vi "PXI Compute Skip Samples.vi"(0 "AO Tasks":T1[](array[typedef]), 7 "AI Tasks":T1[](array[typedef]), 11 "error in (no error)":errorcluster) -> (4 "Skip Samples":i32, 15 "error out":errorcluster)   [LabVIEW 2020]
doc: "Determines the number of AI samples to skip in order to register AO and AI (accounting for the latencies of the 24-bit boards)."
uses:
  Type Defs/Task Struct.ctl
  PXI Globals.vi
panel:
  out "Any 16-bit AI?":bool
  out "Any 16-bit AO?":bool
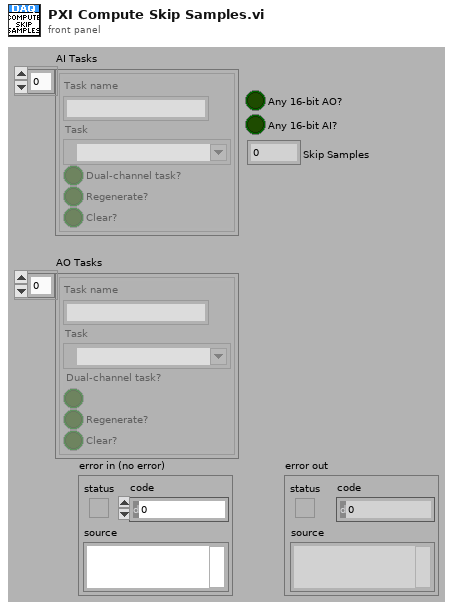
[diagram p1: front panel]
types:
  T1 = typedef "Task Struct.ctl" = cluster{"Task name":string, "Task":refnum<k21>, "Dual-channel task?":bool, "Regenerate?":bool, "Clear?":bool}
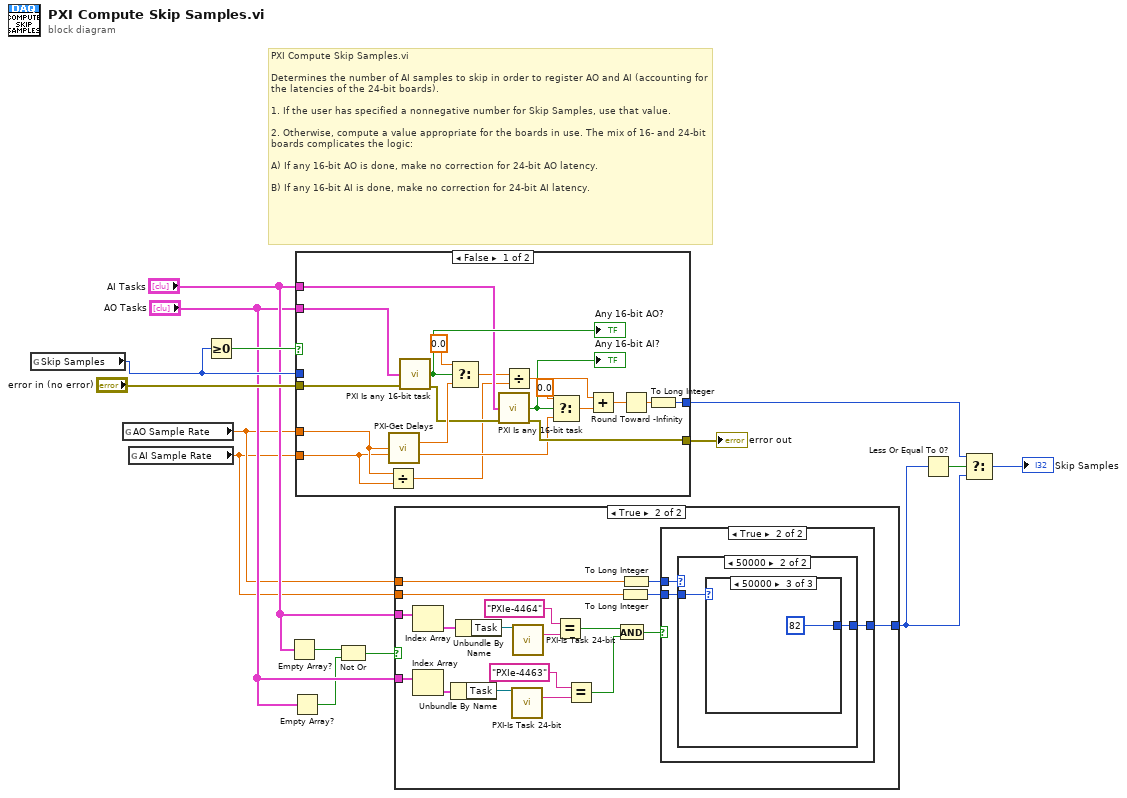
[diagram p0: block diagram]
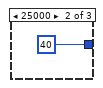
[diagram p6: hidden frame]
diagram:
  # "PXI Compute Skip Samples.vi\n\nDetermines the number of AI samples to skip in order to register AO and AI (accounting for the latencies of the 24-bit boards). \n\n1. If the user has specified a nonnegative number for Skip Samples, use that value. \n\n2. Otherwise, compute a value appropriate for the boards in use. The mix of 16- and 24-bit boards complicates the logic:\n\nA) If any 16-bit AO is done, make no correction for 24-bit AO latency.\n\nB) If any 16-bit AI is done, make no correction for 24-bit AI latency."
  n1 = global read "PXI Globals.vi" "Skip Samples"() -> (w12:i32)
  n2 = global read "PXI Globals.vi" "AO Sample Rate"() -> (w6:dbl)
  n3 = global read "PXI Globals.vi" "AI Sample Rate"() -> (w5:dbl)
  n4 = Greater Or Equal To 0?(x=w12) -> (x >= 0?=w15:bool)
  n5 = Empty Array?(array="AI Tasks") -> (empty?=w9:bool)
  n6 = Empty Array?(array="AO Tasks") -> (empty?=w8:bool)
  n7 = case shown="False" w15 {
    tunnel: "error in (no error)" -> [w16 w37]
    tunnel: [w33 w36] -> w4
    tunnel: [w26 w37] -> w14
    tunnel: w12 -> [_ w36]
    tunnel: "AO Tasks" -> [w32 _]
    tunnel: "AI Tasks" -> [w27 _]
    tunnel: w6 -> [w18 _]
    tunnel: w5 -> [w17 _]
    frame False {
      n8 = Divide(x=w18, y=w17) -> (x/y=w19:dbl)
      n9 = call "PXI-Get Delays.vi"("AO Rate (Samples/s)"=w18, "AI Rate (Samples/s)"=w17) -> ("AO delay (samples)"=w29:dbl, "AI delay (samples)"=w24:dbl)  [unwired: 12 in]
      n10 = call "PXI Is any 16-bit task.vi"("Task Array"=w32, "error in (no error)"=w16) -> ("Any 16-bit task?"=w31:bool, "error out"=w28:errorcluster)  [unwired: 12 in]
      "Any 16-bit AO?" <- w31
      n11 = Select(t=0.0 ("f"), s=w31, f=w29) -> (s? t:f=w21:dbl)
      n12 = call "PXI Is any 16-bit task.vi"("Task Array"=w27, "error in (no error)"=w28) -> ("Any 16-bit task?"=w25:bool, "error out"=w26:errorcluster)  [unwired: 12 in]
      "Any 16-bit AI?" <- w25
      n13 = Divide(x=w21, y=w19) -> (x/y=w20:dbl)
      n14 = Select(t=0.0, s=w25, f=w24) -> (s? t:f=w22:dbl)
      n15 = Add(x=w20, y=w22) -> (x+y=w34:dbl)
      n16 = Round Toward -Infinity(1:w34) -> (0:w35:dbl)
      n17 = To Long Integer(number=w35) -> (32bit integer=w33:i32)
    }
    frame True {
    }
  }
  "error out" <- w14
  n18 = Not Or(1:w8, 2:w9) -> (0:w7:bool)
  n19 = case shown="True" w7 {
    tunnel: "AI Tasks" -> [_ w50]
    tunnel: "AO Tasks" -> [_ w49]
    tunnel: w6 -> [_ w45]
    tunnel: w5 -> [_ w43]
    tunnel: [_ w38] -> w2
    frame False {
    }
    frame True {
      n20 = Index Array(array=w50) -> (element=w55:T1)  [unwired: 1 in]
      n21 = Index Array(array=w49) -> (element=w54:T1)  [unwired: 1 in]
      n22 = Unbundle By Name(w54) -> ("Task"=w51:refnum<k21>)
      n23 = Unbundle By Name(w55) -> ("Task"=w53:refnum<k21>)
      n24 = call "PXI-Is Task 24-bit.vi"("task"=w51) -> ("Product Type"=w39:string)  [unwired: 9 in, 5 out]
      n25 = call "PXI-Is Task 24-bit.vi"("task"=w53) -> ("Product Type"=w40:string)  [unwired: 9 in, 5 out]
      n26 = Equal?(x="PXIe-4464", y=w40) -> (x = y?=w47:bool)
      n27 = Equal?(x="PXIe-4463", y=w39) -> (x = y?=w46:bool)
      n28 = And(x=w47, y=w46) -> (x .and. y?=w41:bool)
      n29 = To Long Integer(number=w43) -> (32bit integer=w42:i32)
      n30 = To Long Integer(number=w45) -> (32bit integer=w44:i32)
      n31 = case shown="True" w41 {
        tunnel: w44 -> [_ w58]
        tunnel: w42 -> [_ w57]
        tunnel: [_ w56] -> w38
        frame False {
        }
        frame True {
          n32 = case shown="50000" w58 {
            tunnel: w57 -> [_ w60]
            tunnel: [_ w59] -> w56
            frame 0, Default {
            }
            frame 50000 {
              n33 = case shown="50000" w60 {
                tunnel: [_ 40 82] -> w59
                frame 0, Default {
                }
                frame 25000 {
                }
                frame 50000 {
                }
              }
            }
          }
        }
      }
    }
  }
  n34 = Less Or Equal To 0?(x=w2) -> (x <= 0?=w1:bool)
  n35 = Select(t=w4, s=w1, f=w2) -> (s? t:f=→"Skip Samples":i32)
